vi "disk_zipDiskTemplate.vi"(8 "error in (no error)":errorcluster, 10 "template tail":string[](array[string]), 11 "DiskTemplate in":T1={"XMLRef"=[refnum, refnum, refnum, refnum, refnum, refnum], "ZipPath"=path "", "MetaFile"={"Ref"=refnum, "NextRow"=0, "NextPosition"=0, "Block"=[]}, "TempFolder"=path ""}) -> (0 "error out":errorcluster, 3 "DiskTemplate out":T1)   [LabVIEW 2017, in "NI_ExcelFile.lvlib"]
uses:
  <vilib>/express/express shared/NI_ExcelFile/NI_ExcelFile.lvlib
  <vilib>/express/express shared/NI_ExcelFile/Ctrls/disk_TemplateFile.ctl
  <vilib>/express/express shared/NI_ExcelFile/Ctrls/meta_file.ctl
  <vilib>/express/express shared/NI_ExcelFile/Ctrls/meta_Block.ctl
  <vilib>/express/express shared/NI_ExcelFile/Ctrls/meta_BlockType.ctl
  <vilib>/express/express shared/NI_ExcelFile/Ctrls/TemplateEnum.ctl
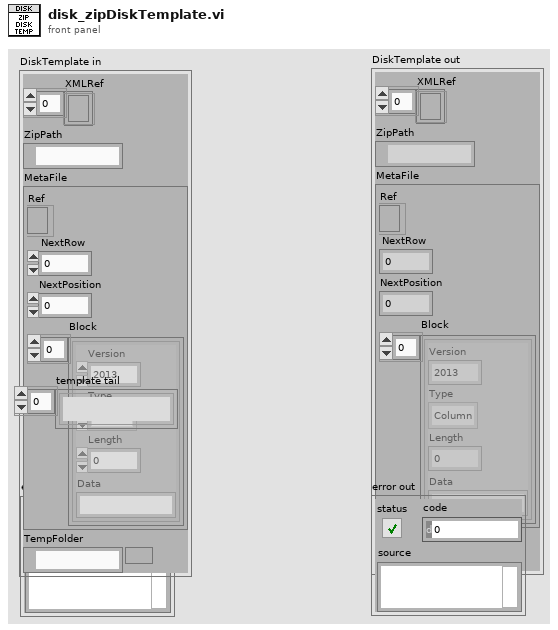
[diagram p1: front panel]
types:
  T1 = typedef "NI_ExcelFile.lvlib/disk_TemplateFile.ctl" = cluster{"XMLRef":refnum<file>[], "ZipPath":path, "MetaFile":T2, "TempFolder":path}
  T2 = typedef "NI_ExcelFile.lvlib/meta_file.ctl" = cluster{"Ref":refnum<file>, "NextRow":i32, "NextPosition":i64, "Block":T3[]}
  T3 = typedef "NI_ExcelFile.lvlib/meta_Block.ctl" = cluster{"Version":u16, "Type":T4, "Length":i32, "Data":string}
  T4 = typedef "NI_ExcelFile.lvlib/meta_BlockType.ctl" = enum16{"NITag", "File", "Column"}
  T5 = typedef "NI_ExcelFile.lvlib/TemplateEnum.ctl" = enum16{"[Content_Types].xml", ".rels", "workbook.xml", "styles.xml", "workbook.xml.rels", "sheet.xml", "app.xml", "core.xml"}
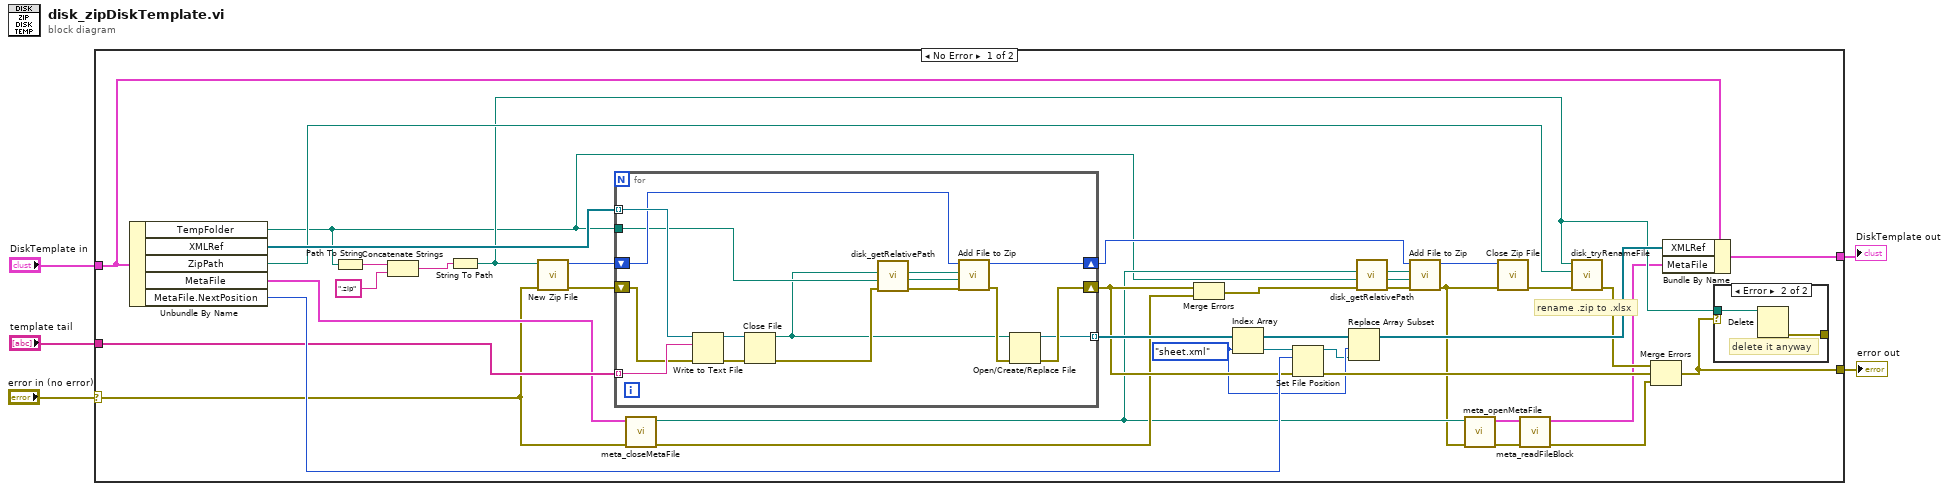
[diagram p0: block diagram]
diagram:
  n1 = case shown="No Error" "error in (no error)" {
    selector: "error in (no error)" -> [w14 w63]
    tunnel: "DiskTemplate in" -> [w43 w64]
    tunnel: [w42 w64] -> w4
    tunnel: [w24 w63] -> w1
    tunnel: "template tail" -> [w26 _]
    frame No Error {
      w23 = TemplateEnum."sheet.xml" ("Template")
      # "rename .zip to .xlsx"
      n2 = Unbundle By Name(w43) -> ("TempFolder"=w6:path, "XMLRef"=w34:refnum<file>[], "ZipPath"=w33:path, "MetaFile"=w15:T2, "MetaFile.NextPosition"=w30:i64)
      n3 = Path To String(path=w6) -> (string=w38:string)
      n4 = Concatenate Strings(w38, ".zip") -> (w37:string)
      n5 = String To Path(string=w37) -> (path=w25:path)
      n6 = call <vilib>:"New Zip File.vi"("error in (no error)"=w14, "target"=w25) -> ("error out"=w40:errorcluster, "zip file out"=w41:i64)  [unwired: 3 in, 1 out]
      n7 = for {
        tunnel: w34 -> [w61] mode=indexing
        tunnel: w26 -> [w59] mode=indexing
        shift-right: [w54] -> w27
        shift-left: w40 -> [w56]
        shift-right: [w58] -> w16
        shift-left: w41 -> [w57]
        tunnel: w6 -> [w48]
        tunnel: [w53] -> w32 mode=indexing
        n8 = Write to Text File(file (use dialog)=w61, text=w59, error in=w56) -> (refnum out=w60:refnum<file>, error out=w62:errorcluster)  [unwired: 1 in, 1 out]
        n9 = Close File(refnum=w60, error in=w62) -> (path=w47:path, error out=w49:errorcluster)
        n10 = call <vilib>:"disk_getRelativePath.vi"("error in (no error)"=w49, "temp folder"=w48, "absolute path"=w47) -> ("error out"=w50:errorcluster, "relative path out"=w51:path, "absolute path out"=w52:path)  [unwired: 6 in]
        n11 = call <vilib>:"Add File to Zip.vi"("error in (no error)"=w50, "destination path in zip"=w51, "source file path"=w52, "zip file in"=w57) -> ("error out"=w55:errorcluster, "zip file out"=w58:i64)  [unwired: 6 in]
        n12 = Open/Create/Replace File(file path (use dialog)=w47, error in=w55) -> (refnum out=w53:refnum<file>, error out=w54:errorcluster)  [unwired: 4 in, 1 out]
      }
      n13 = call <vilib>:"meta_closeMetaFile.vi"("error in (no error)"=w14, "meta file in"=w15) -> ("error out"=w13:errorcluster, "path"=w12:path)  [unwired: 8 in]
      n14 = Merge Errors(w27, w13) -> (w17:errorcluster)
      n15 = Index Array(array=w32, index=w23) -> (element=w22:refnum<file>)
      n16 = Set File Position(offset (in bytes) (0)=w30, refnum=w22, error in=w27) -> (refnum out=w21:refnum<file>, error out=w28:errorcluster)  [unwired: 1 in]
      n17 = Replace Array Subset(array=w32, new element=w21, index=w23) -> (w31:refnum<file>[])
      n18 = call <vilib>:"disk_getRelativePath.vi"("error in (no error)"=w17, "temp folder"=w6, "absolute path"=w12) -> ("error out"=w20:errorcluster, "relative path out"=w19:path, "absolute path out"=w18:path)  [unwired: 6 in]
      n19 = call <vilib>:"Add File to Zip.vi"("error in (no error)"=w20, "destination path in zip"=w19, "source file path"=w18, "zip file in"=w16) -> ("error out"=w11:errorcluster, "zip file out"=w39:i64)  [unwired: 6 in]
      n20 = call <vilib>:"meta_openMetaFile.vi"("error in"=w11, "path"=w12) -> ("error out"=w10:errorcluster, "meta file"=w9:T2)  [unwired: 8 in]
      n21 = call <vilib>:"Close Zip File.vi"("error in (no error)"=w11, "zip file in"=w39) -> ("error out"=w35:errorcluster)  [unwired: 5 in]
      n22 = call <vilib>:"meta_readFileBlock.vi"("error in (no error)"=w10, "meta file in"=w9) -> ("error out"=w8:errorcluster, "meta file out"=w7:T2)  [unwired: 7 in, 1 out]
      n23 = call <vilib>:"disk_tryRenameFile.vi"("error in (no error)"=w35, "target path"=w33, "source path"=w25) -> ("error out"=w29:errorcluster)  [unwired: 8 in]
      n24 = Merge Errors(w29, w28, w8) -> (w24:errorcluster)
      n25 = Bundle By Name(cluster=w43, "XMLRef"=w31, "MetaFile"=w7) -> (w42:T1)
      n26 = case shown="Error" w24 {
        selector: w24 -> [w44 _]
        tunnel: w25 -> [_ w46]
        tunnel: [w44 w45] -> _
        frame No Error {
        }
        frame Error {
          # "delete it anyway"
          n27 = Delete(path (use dialog)=w46) -> (error out=w45:errorcluster)  [unwired: 4 in, 2 out]
        }
      }
    }
    frame Error {
    }
  }
  "DiskTemplate out" <- w4
  "error out" <- w1
